vi "AnnexDSim.vi"(8 "error in (no error)":errorcluster, 11 "C37.118 Sim in":refnum<class "C37.118 Sim.lvclass">) -> (0 "error out":errorcluster, 3 "C37.118 Sim out":refnum<class "C37.118 Sim.lvclass">)   [LabVIEW 2014, in "SensorPlugins.lvlib" / "C37.118 Sim.lvclass"]
uses:
  C37.118 Sim.lvclass
  C37.118 Sim.lvclass/C37.118 Sim.ctl
  PmuBaseClass/PmuBase.lvclass/PmuBase.ctl
  PmuBaseClass/Typedef/PmuData.ctl
  Accessors/Read EvtSignal.vi
  PmuBaseClass/Accessors/Read PmuConfig.vi
  PmuBaseClass/Accessors/Write PmuDataArray.vi
  <vilib>/imath/engines/lvmath2/RunTimeEngine/Managers/WorkSpace/UID Generator.vi
  <vilib>/imath/engines/lvmath/Plug In/_Char/NIMS_CH_String to Character Array.vi
  C:/Labview Data/MathScriptVIs/MCStatic_33564263232_179b4987dfd00f1dbab995646ad239b6.vi
  <instcachedir>/0/MCStatic_33564263232_179b4987dfd00f1dbab995646ad239b6_F68478F465BC41CE9228F2FCAB70A875.lvgen/MCStatic_33564263232_179b4987dfd00f1dbab995646ad239b6_F68478F465BC41CE9228F2FCAB70A875_000.vi
  <vilib>/imath/engines/lvmath2/RunTimeEngine/UserFunctionToken/NIMS_UserFunction_CondDefined.vi
  <instcachedir>/0/NIMS_UserFunction_CondDefined_359D6D699583402F98E5D4DB7FB40D41.lvgen/NIMS_UserFunction_CondDefined_359D6D699583402F98E5D4DB7FB40D41_000.vi
  <vilib>/imath/engines/lvmath2/RunTimeEngine/RunTimeType/NIMS_RunTimeType_From StrictType (excl LVString).vi
  <instcachedir>/0/NIMS_RunTimeType_From StrictType (excl LVString)_15A5391EEA9C4AACB9955AC755B83D29.lvgen/NIMS_RunTimeType_From StrictType (excl LVString)_15A5391EEA9C4AACB9955AC755B83D29_000.vi
  <instcachedir>/0/NIMS_UserFunction_CondDefined_359D6D699583402F98E5D4DB7FB40D41.lvgen/NIMS_UserFunction_CondDefined_359D6D699583402F98E5D4DB7FB40D41_001.vi
  <instcachedir>/0/NIMS_UserFunction_CondDefined_359D6D699583402F98E5D4DB7FB40D41.lvgen/NIMS_UserFunction_CondDefined_359D6D699583402F98E5D4DB7FB40D41_003.vi
  <vilib>/imathl/engines/lvmath/Functions/Error Handling/Create Error.vi
  <vilib>/imath/engines/lvmath2/RunTimeEngine/LocalVariableDefStatement/MC_LocalVariableDefStatement_Display.vi
  <vilib>/imath/engines/lvmath2/RunTimeEngine/VariableToken/NIMS_VariableToken_CondDefined.vi
  <instcachedir>/0/NIMS_VariableToken_CondDefined_EE8DD211A89249938CE6537267F5C9B3.lvgen/NIMS_VariableToken_CondDefined_EE8DD211A89249938CE6537267F5C9B3_003.vi
  <instcachedir>/0/NIMS_VariableToken_CondDefined_EE8DD211A89249938CE6537267F5C9B3.lvgen/NIMS_VariableToken_CondDefined_EE8DD211A89249938CE6537267F5C9B3_002.vi
  <instcachedir>/0/NIMS_VariableToken_CondDefined_EE8DD211A89249938CE6537267F5C9B3.lvgen/NIMS_VariableToken_CondDefined_EE8DD211A89249938CE6537267F5C9B3_004.vi
  <vilib>/imath/engines/lvmath/Functions/Error Handling/MergeErrorsWrapper.vi
  <vilib>/imath/engines/lvmath2/RunTimeEngine/Managers/SymbolTable/Clear UID.vi
  <vilib>/imath/engines/lvmath2/RunTimeEngine/NodeEndStatement/NIMS_NodeEndStatement_Output.vi
  <instcachedir>/0/NIMS_NodeEndStatement_Output_53EC0D466D134D7ABD903AC30B43404B.lvgen/NIMS_NodeEndStatement_Output_53EC0D466D134D7ABD903AC30B43404B_017.vi
  <instcachedir>/0/NIMS_NodeEndStatement_Output_53EC0D466D134D7ABD903AC30B43404B.lvgen/NIMS_NodeEndStatement_Output_53EC0D466D134D7ABD903AC30B43404B_003.vi
  <instcachedir>/0/NIMS_NodeEndStatement_Output_53EC0D466D134D7ABD903AC30B43404B.lvgen/NIMS_NodeEndStatement_Output_53EC0D466D134D7ABD903AC30B43404B_005.vi
  <vilib>/imath/engines/lvmath2/RunTimeEngine/ErrorHandling/NIMS_Finalize Error.vi
  Matlab/AnnexDPmu.m
  Matlab/blackman.m
  Matlab/calcPosSeq.m
  Matlab/FIR.m
  Matlab/hamming.m
  Matlab/hann.m
  Matlab/Window.m
  PmuBaseClass/PmuBase.lvclass
  <vilib>/imath/engines/lvmath2/RunTimeEngine/Managers/SymbolTable/NIMS_WorkSpace.lvlib
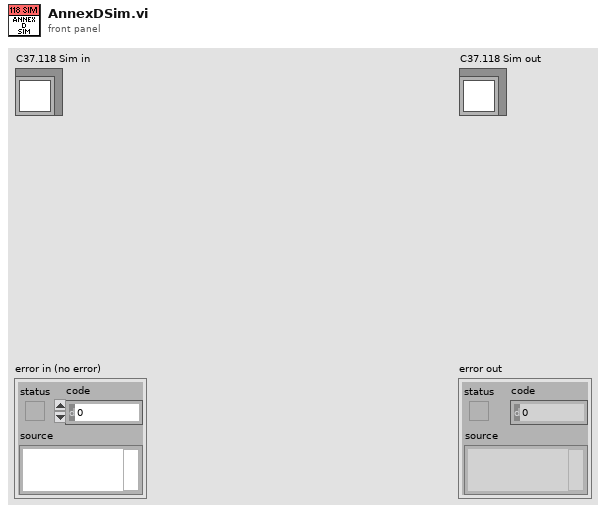
[diagram p1: front panel]
types:
  T1 = typedef "SensorPlugins.lvlib/PmuBase.lvclass/PmuData.ctl" = cluster{"Timestamp":dbl, "Synx":cdb[], "Freq":dbl, "ROCOF":dbl, "ID":i16}
  T2 = typedef "SensorPlugins.lvlib/PmuBase.lvclass/PmuConfig.ctl" = cluster{"Class":enum16{"M", "P"}, "Fs":i32, "F0":i32, "FSamp":i32, "SettlingTime":dbl, "T0":ext}
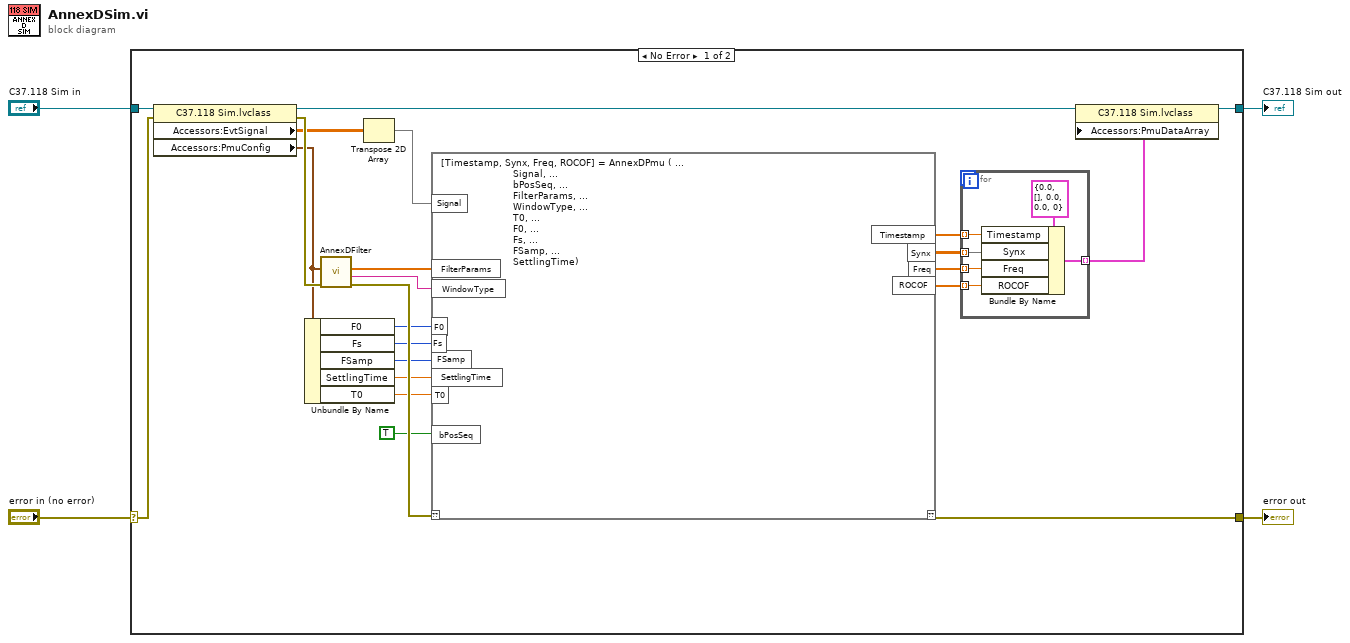
[diagram p0: block diagram]
diagram:
  n1 = case shown="No Error" "error in (no error)" {
    selector: "error in (no error)" -> [w25 w232]
    tunnel: [w13 w232] -> w3
    tunnel: [w8 w231] -> w1
    tunnel: "C37.118 Sim in" -> [w26 w231]
    frame No Error {
      n2 = property class="C37.118 Sim.lvclass"(reference=w26, error in=w25) -> (reference out=w27:refnum<class "C37.118 Sim.lvclass">, error out=w24:errorcluster, "Accessors:EvtSignal"=w23:dbl[][], "Accessors:PmuConfig"=w22:T2)
      n3 = Unbundle By Name(w22) -> ("F0"=w16:i32, "Fs"=w15:i32, "FSamp"=w14:i32, "SettlingTime"=w18:dbl, "T0"=w5:ext)
      n4 = call "AnnexDFilter.vi"("error in (no error)"=w24, "PmuConfig"=w22) -> ("error out"=w19:errorcluster, "WindowType"=w20:string, "FilterParams"=w21:dbl[])  [unwired: 7 in]
      n5 = Transpose 2D Array(2D array=w23) -> (transposed array=w6:dbl[][])
      n6 = mathscript code="[Timestamp, Synx, Freq, ROCOF] = AnnexDPmu ( ...\n                        Signal, ...\n                        bPosSeq, ...\n                        FilterParams, ...\n                        WindowType, ...\n                        T0, ...\n                        F0, ...\n                        Fs, ...\n                        FSamp, ...\n                        SettlingTime)"("??"=w19, "Signal"=w6, "T0"=w5, "FilterParams"=w21, "WindowType"=w20, "SettlingTime"=w18, "FSamp"=w14, "bPosSeq"=TRUE, "F0"=w16, "Fs"=w15) -> ("??"=w13:errorcluster, "Freq"=w11:dbl[], "ROCOF"=w10:dbl[], "Synx"=w9:cdb[][], "Timestamp"=w12:ext[])
      n7 = for {
        tunnel: w12 -> [w33] mode=indexing
        tunnel: w11 -> [w31] mode=indexing
        tunnel: w10 -> [w30] mode=indexing
        tunnel: w9 -> [w32] mode=indexing
        tunnel: [w29] -> w7 mode=indexing
        n8 = Bundle By Name(cluster=T1 {"Timestamp"=0.0, "Synx"=[], "Freq"=0.0, "ROCOF"=0.0, "ID"=0} ("PmuReport"), "Timestamp"=w33, "Synx"=w32, "Freq"=w31, "ROCOF"=w30) -> (w29:T1)
      }
      n9 = property class="C37.118 Sim.lvclass"(reference=w27, "Accessors:PmuDataArray"=w7) -> (reference out=w8:refnum<class "C37.118 Sim.lvclass">)  [unwired: 1 in, 1 out]
    }
    frame Error {
    }
  }
  "error out" <- w3
  "C37.118 Sim out" <- w1
